vi "Refname to String (Controllers).vi"(1 "Enum":T1) -> (0 "string":string)   [LabVIEW 2016]
uses:
  Controllers.ctl
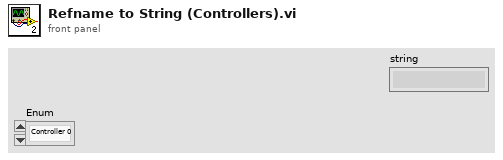
[diagram p1: front panel]
types:
  T1 = typedef "Controllers.ctl" = enum16{"Controller 0", "Controller 1"}
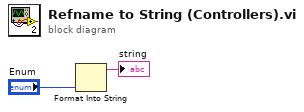
[diagram p0: block diagram]
diagram:
  n1 = Format Into String("Enum") -> (resulting string=→"string":string)  [unwired: 3 in, 1 out]
